vi "upload_details_from_spreadsheet.vi"(11 "Upload Spreadsheet path":path) -> (3 "Device details":T1={"Cell Position"=1, "Cell Label"="", "Pixel to measure"=0, "Area (cm^2)"=0.0919, "Variable"="", "Variable value"="", "Scan settings"=0} {"Pixel to measure" items=["All", "1", "2", "3", "4", "5", "6", "7", "8"]})   [LabVIEW 2016]
uses:
  <vilib>/Utility/file.llb/Read Delimited Spreadsheet (string).vi
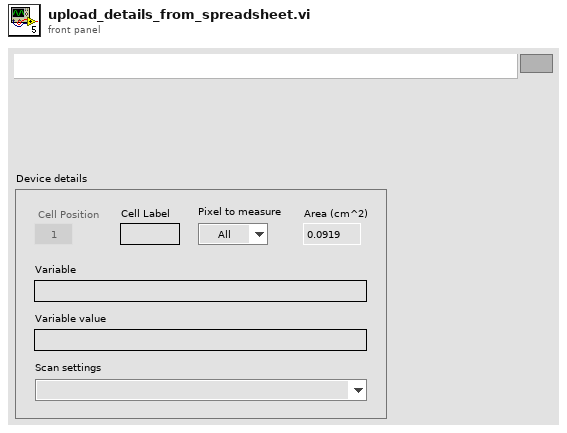
[diagram p1: front panel]
types:
  T1 = cluster{"Cell Position":i32, "Cell Label":string, "Pixel to measure":u16, "Area (cm^2)":dbl, "Variable":string, "Variable value":string, "Scan settings":u16}
  T2 = cluster{"Cell Position":i32, "Cell Label":string, "Pixel to measure":u16, "Area (cm^2)":dbl, "Variable":string, "Variable value":string, "Scan settings in queue":u16}
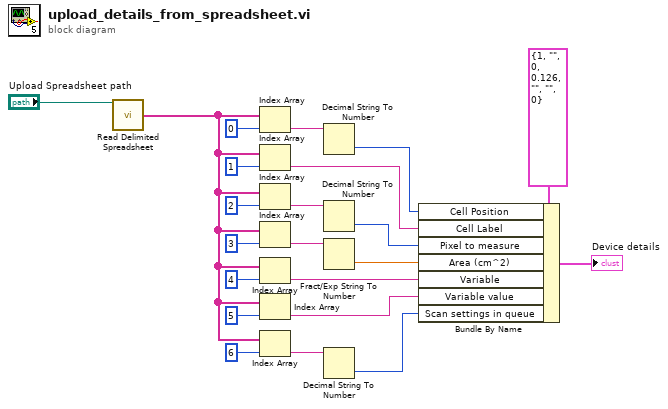
[diagram p0: block diagram]
diagram:
  n1 = call-poly <vilib>:"Read Delimited Spreadsheet.vi"("file path (dialog if empty)"="Upload Spreadsheet path") -> ("first row"=w2:string[])  [unwired: 9 in, 5 out]
  n2 = Index Array(array=w2, index=0) -> (element=w13:string)
  n3 = Index Array(array=w2, index=1) -> (element=w11:string)
  n4 = Index Array(array=w2, index=2) -> (element=w10:string)
  n5 = Index Array(array=w2, index=3) -> (element=w9:string)
  n6 = Index Array(array=w2, index=4) -> (element=w7:string)
  n7 = Index Array(array=w2, index=5) -> (element=w6:string)
  n8 = Index Array(array=w2, index=6) -> (element=w5:string)
  n9 = Decimal String To Number(string=w13) -> (number=w12:i32)  [unwired: 2 in, 1 out]
  n10 = Decimal String To Number(string=w10) -> (number=w3:i32)  [unwired: 2 in, 1 out]
  n11 = Fract/Exp String To Number(string=w9) -> (number=w8:dbl)  [unwired: 3 in, 1 out]
  n12 = Decimal String To Number(string=w5) -> (number=w4:i32)  [unwired: 2 in, 1 out]
  n13 = Bundle By Name(cluster=T2 {"Cell Position"=1, "Cell Label"="", "Pixel to measure"=0, "Area (cm^2)"=0.126, "Variable"="", "Variable value"="", "Scan settings in queue"=0} ("System Cluster"), "Cell Position"=w12, "Cell Label"=w11, "Pixel to measure"=w3, "Area (cm^2)"=w8, "Variable"=w7, "Variable value"=w6, "Scan settings in queue"=w4) -> (→"Device details":T2)
